vi "DataLogging_v2.vi"(4 "Tab?":bool, 6 "New Line?":bool, 7 "Name":string, 8 "error in (no error)":errorcluster, 10 "WriteToFile?":bool, 11 "Variant In":variant) -> (0 "error out":errorcluster, 3 "FinalText":string)   [LabVIEW 2017]
uses:
  <vilib>/Utility/Data Type/Type Definitions/Data Type.ctl
  <vilib>/Utility/Data Type/NI_Data Type.lvlib
panel:
  out "Type":T1
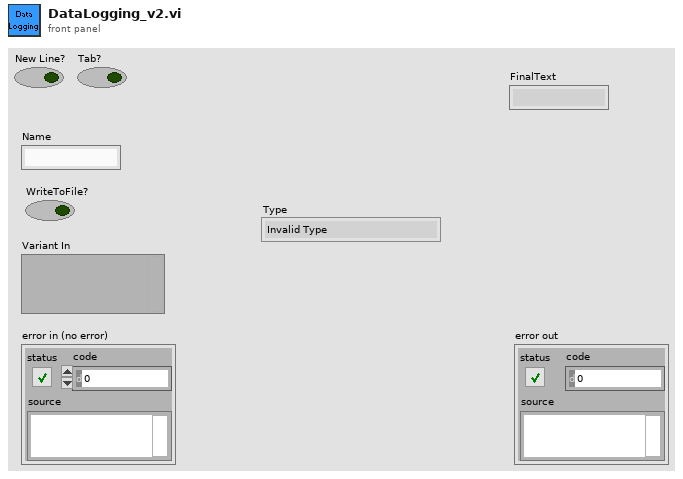
[diagram p1: front panel]
types:
  T1 = typedef "NI_Data Type.lvlib/Data Type.ctl" = enum8{"Invalid Type", "Void", "I8", "I16", "I32", "I64", "U8", "U16", "U32", "U64", "Single Float", "Double Float", "Extended Float", "Single Complex", "Double Complex", "Extended Complex", "Enum U8", "Enum U16", "Enum U32", "Enum U64", "Single Float With Unit", "Double Float With Unit", "Extended Float With Unit", "Single Complex with Unit", "Double Complex with Unit", "Extended Complex with Unit", "Boolean", "String", "Path", "Picture", "Tag", "Array", "Cluster", "Variant", "LV Variant", "Waveform", "Timestamp", "Digital Waveform", "Digital Data", "ExpressData", "Refnum", "External Data", "VI", "Poly VI", "LabVIEW Class Instance", "Fixed Point"}
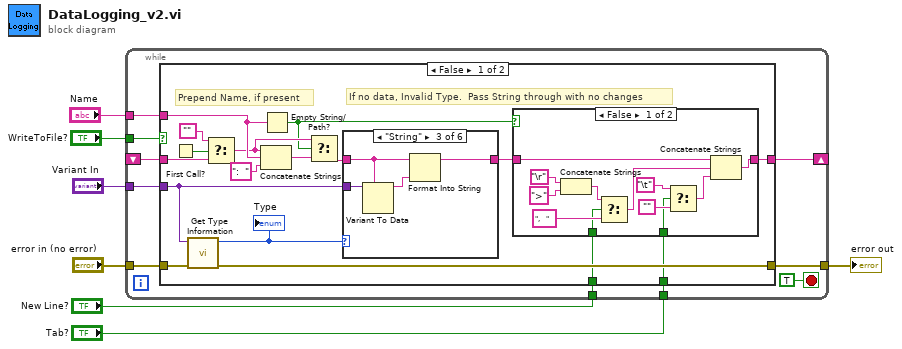
[diagram p0: block diagram]
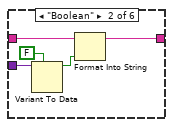
[diagram p4: hidden frame]
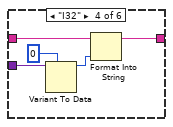
[diagram p5: hidden frame]
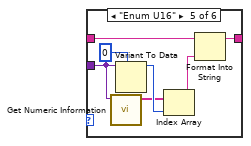
[diagram p6: hidden frame]
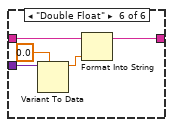
[diagram p7: hidden frame]
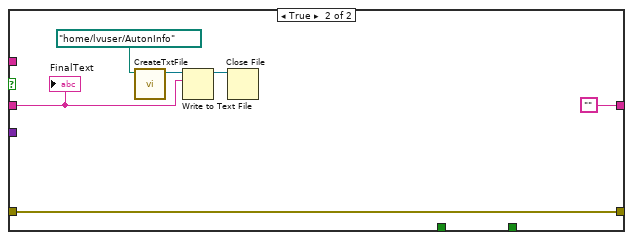
[diagram p8: hidden frame]
diagram:
  n1 = while {
    tunnel: "Variant In" -> [w17]
    shift-right: [w10] -> _
    shift-left: _ -> [w13]
    tunnel: "WriteToFile?" -> [w8]
    tunnel: "error in (no error)" -> [w15]
    tunnel: [w14] -> w4
    tunnel: "Name" -> [w12]
    tunnel: "New Line?" -> [w11]
    tunnel: "Tab?" -> [w9]
    stop <- TRUE stop-if-true
    n2 = case shown="False" w8 {
      tunnel: w17 -> [w34 _]
      tunnel: w15 -> [w33 w80]
      tunnel: [w32 w80] -> w14
      tunnel: w13 -> [w19 w77]
      tunnel: w12 -> [w29 _]
      tunnel: w11 -> [w24 _]
      tunnel: [w20 ""] -> w10
      tunnel: w9 -> [w22 _]
      frame False {
        # "If no data, Invalid Type.  Pass String through with no changes"
        # "Prepend Name, if present"
        n3 = First Call?() -> (First Call?: T/F=w30:bool)
        n4 = call <vilib>:"Get Type Information.vi"("error in (no error)"=w33, "Variant"=w34) -> ("error out"=w32:errorcluster, "Type"=w21:T1)  [unwired: 5 in, 3 out]
        "Type" <- w21
        n5 = Select(t="", s=w30, f=w19) -> (s? t:f=w26:string)
        n6 = Concatenate Strings(w26, w29, ":  " ("string")) -> (w27:string)
        n7 = Empty String/Path?(string/path=w29) -> (empty?=w18:bool)
        n8 = Select(t=w26, s=w18, f=w27) -> (s? t:f=w28:string)
        n9 = case shown="\"String\"" w21 {
          tunnel: w34 -> [_ w53 w57 w62 w65 w72]
          tunnel: [w48 w50 w55 w60 w69 w74] -> w23
          tunnel: w28 -> [w48 w49 w54 w59 w68 w73]
          frame "Invalid Type", Default {
          }
          frame "Boolean" {
            n10 = Variant To Data(type=FALSE, Variant=w53) -> (data=w51:bool)  [unwired: 1 in, 1 out]
            n11 = Format Into String(initial string=w49, w51) -> (resulting string=w50:string)  [unwired: 2 in, 1 out]
          }
          frame "String" {
            n12 = Variant To Data(type=w54, Variant=w57) -> (data=w56:string)  [unwired: 1 in, 1 out]
            n13 = Format Into String(initial string=w54, w56) -> (resulting string=w55:string)  [unwired: 2 in, 1 out]
          }
          frame "I32" {
            n14 = Variant To Data(type=0, Variant=w62) -> (data=w61:i32)  [unwired: 1 in, 1 out]
            n15 = Format Into String(initial string=w59, w61) -> (resulting string=w60:string)  [unwired: 2 in, 1 out]
          }
          frame "Enum U16" {
            n16 = call <vilib>:"Get Numeric Information.vi"("Variant"=w65) -> ("Enum Names"=w66:string[])  [unwired: 7 in, 3 out]
            n17 = Variant To Data(type=0, Variant=w65) -> (data=w67:i32)  [unwired: 1 in, 1 out]
            n18 = Index Array(array=w66, index=w67) -> (element=w64:string)
            n19 = Format Into String(initial string=w68, w64) -> (resulting string=w69:string)  [unwired: 2 in, 1 out]
          }
          frame "Double Float" {
            n20 = Variant To Data(type=0.0, Variant=w72) -> (data=w70:dbl)  [unwired: 1 in, 1 out]
            n21 = Format Into String(initial string=w73, w70) -> (resulting string=w74:string)  [unwired: 2 in, 1 out]
          }
        }
        n22 = case shown="False" w18 {
          tunnel: w24 -> [w43 _]
          tunnel: w23 -> [w42 w47]
          tunnel: w22 -> [w36 _]
          tunnel: [w35 w47] -> w20
          frame False {
            n23 = Concatenate Strings("\r", ">") -> (w44:string)
            n24 = Select(t=w44, s=w43, f=",   ") -> (s? t:f=w41:string)
            n25 = Select(t="\t", s=w36, f="") -> (s? t:f=w39:string)
            n26 = Concatenate Strings(w42, w41, w39) -> (w35:string)
          }
          frame True {
          }
        }
      }
      frame True {
        n27 = call "CreateTxtFile.vi"("pathIn"=path "/home/lvuser/AutonInfo") -> ("refnumOut"=w78:refnum<file>)  [unwired: 10 in]
        n28 = Write to Text File(file (use dialog)=w78, text=w77) -> (refnum out=w79:refnum<file>)  [unwired: 2 in, 2 out]
        n29 = Close File(refnum=w79) -> ()  [unwired: 1 in, 2 out]
        "FinalText" <- w77
      }
    }
  }
  "error out" <- w4
